vi "Main.vi"   [LabVIEW 2014]
uses:
  CRDS/Main/eCRDS.lvclass
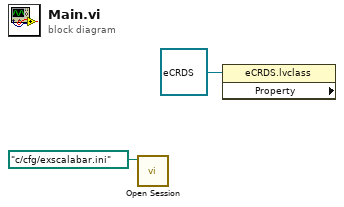
[diagram p0: block diagram]
diagram:
  n1 = call "Open Session.vi"("Path"=path "c:/cfg/exscalabar.ini") -> ()  [unwired: 9 in, 2 out]
  n2 = property class="eCRDS.lvclass" props=[](reference=refnum<class "eCRDS.lvclass"> refnum ("eCRDS")) -> ()  [unwired: 1 in, 3 out]
